vi "ZCP filiter.vi"(2 "Cutoff Frequency":i32=100, 3 "Sampling Frequency":i32=200000, 4 "Noise Band":dbl=-2.0, 5 "Data":dbl[](array[numeric])) -> (0 "Filiter Voltage":dbl[](array[numeric]), 1 "ZCP":i32[](array[numeric]))   [LabVIEW 2013]
uses:
  <vilib>/ptbypt/NI_PtbyPt.lvlib
panel:
  out "Waveform Graph":dbl[][](graph)
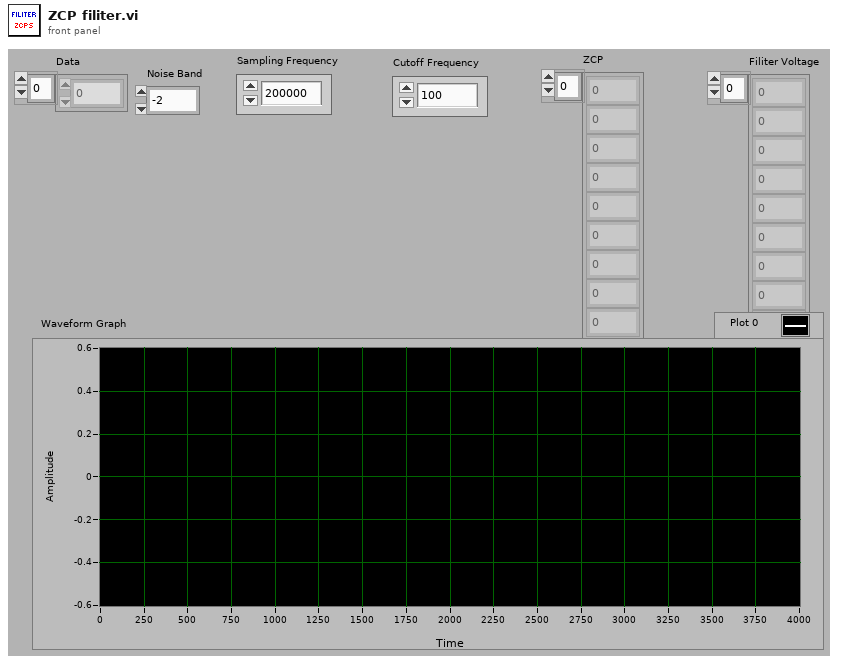
[diagram p1: front panel]
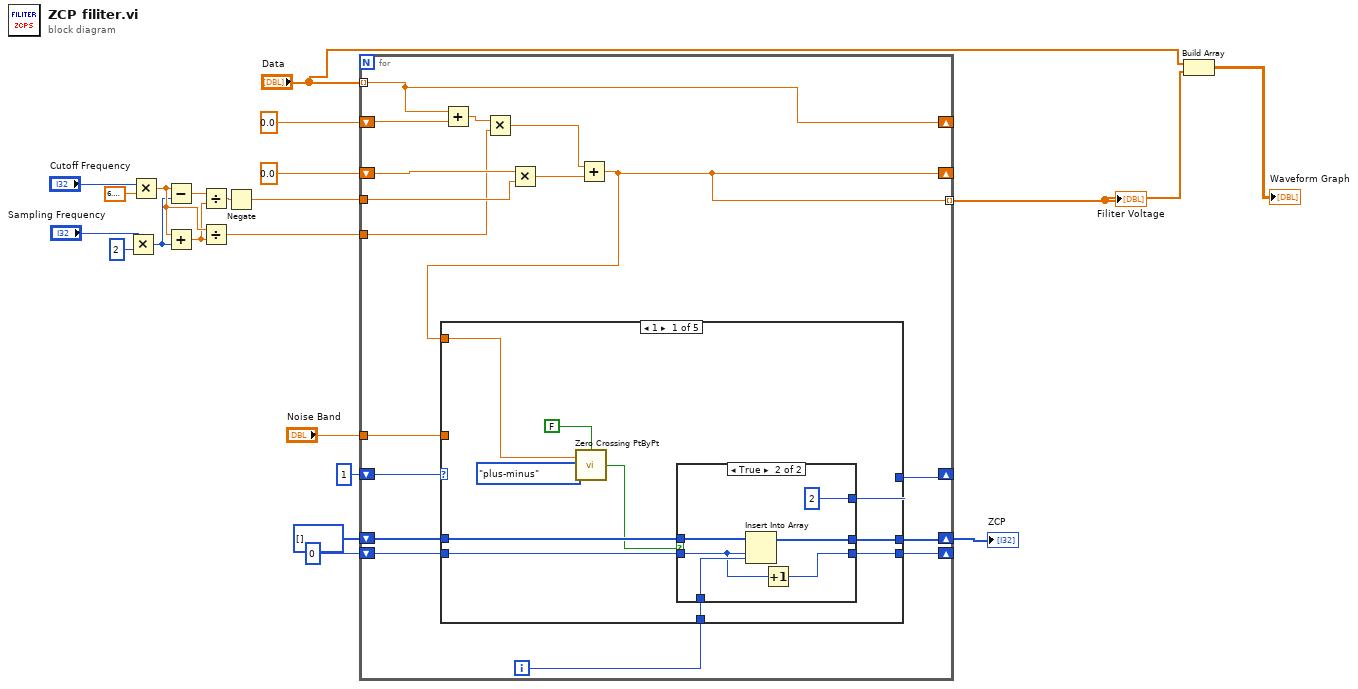
[diagram p0: block diagram]
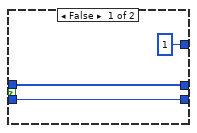
[diagram p2: hidden frame]
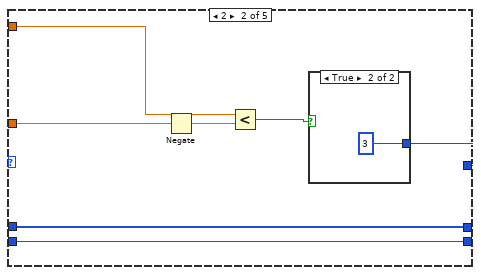
[diagram p3: hidden frame]
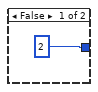
[diagram p4: hidden frame]
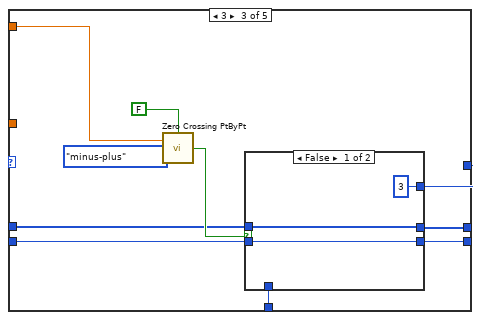
[diagram p5: hidden frame]
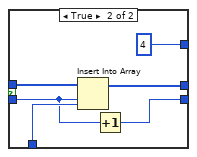
[diagram p6: hidden frame]
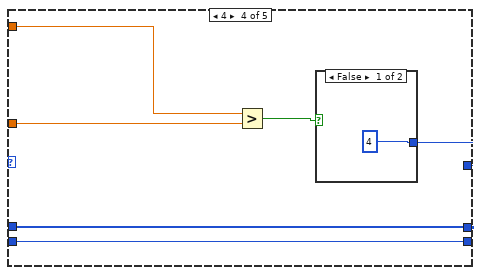
[diagram p7: hidden frame]
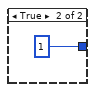
[diagram p8: hidden frame]
diagram:
  n1 = Multiply(x="Sampling Frequency", y=i16 2) -> (x*y=w13:i32)
  n2 = Multiply(x="Cutoff Frequency", y=6.283185307179586) -> (x*y=w14:dbl)
  n3 = Subtract(x=w14, y=w13) -> (x-y=w12:dbl)
  n4 = Add(x=w14, y=w13) -> (x+y=w11:dbl)
  n5 = Divide(x=w12, y=w11) -> (x/y=w8:dbl)
  n6 = Divide(x=w14, y=w11) -> (x/y=w6:dbl)
  n7 = Negate(x=w8) -> (-x=w7:dbl)
  n8 = for {
    shift-right: [w37] -> _
    shift-left: 1 -> [w38]
    tunnel: "Data" -> [w23] mode=indexing
    shift-right: [w34] -> w20
    shift-left: i32[] [] -> [w35]
    shift-right: [w32] -> _
    shift-left: 0 -> [w33]
    tunnel: "Noise Band" -> [w31]
    shift-right: [w23] -> _
    shift-left: 0.0 -> [w30]
    shift-right: [w22] -> _
    shift-left: 0.0 -> [w28]
    tunnel: w7 -> [w27]
    tunnel: w6 -> [w26]
    tunnel: [w22] -> w2 mode=indexing
    i -> [w36]
    n9 = Add(x=w23, y=w30) -> (x+y=w29:dbl)
    n10 = Multiply(x=w29, y=w26) -> (x*y=w25:dbl)
    n11 = Multiply(x=w28, y=w27) -> (x*y=w24:dbl)
    n12 = Add(x=w25, y=w24) -> (x+y=w22:dbl)
    n13 = case shown="1" w38 {
      tunnel: [w39 w60 w67 w87 _] -> w37
      tunnel: w22 -> [w47 w62 w74 w88 _]
      tunnel: w36 -> [w43 _ w68 _ _]
      tunnel: w35 -> [w45 w64 w72 w91 w95]
      tunnel: [w44 w64 w70 w91 w95] -> w34
      tunnel: w33 -> [w42 w63 w71 w90 w94]
      tunnel: [w40 w63 w69 w90 w94] -> w32
      tunnel: w31 -> [_ w59 _ w86 _]
      frame 1 {
        n14 = call <vilib>:"Zero Crossing PtByPt.vi"("initialize"=FALSE, "direction"=enum16{"either", "minus-plus", "plus-minus"}."plus-minus", "input data point"=w47) -> ("crossing"=w41:bool)
        n15 = case shown="True" w41 {
          tunnel: w45 -> [w51 w57]
          tunnel: [w51 w56] -> w44
          tunnel: w43 -> [_ w55]
          tunnel: w42 -> [w50 w54]
          tunnel: [w50 w53] -> w40
          tunnel: [1 2] -> w39
          frame False {
          }
          frame True {
            n16 = Insert Into Array(array=w57, index=w54, new element=w55) -> (w56:i32[])
            n17 = Increment(x=w54) -> (x+1=w53:i32)
          }
        }
      }
      frame 2 {
        n18 = Negate(x=w59) -> (-x=w58:dbl)
        n19 = Less?(x=w62, y=w58) -> (x < y?=w61:bool)
        n20 = case shown="True" w61 {
          tunnel: [2 3] -> w60
          frame False {
          }
          frame True {
          }
        }
      }
      frame 3 {
        n21 = call <vilib>:"Zero Crossing PtByPt.vi"("initialize"=FALSE, "direction"=enum16{"either", "minus-plus", "plus-minus"}."minus-plus", "input data point"=w74) -> ("crossing"=w73:bool)
        n22 = case shown="False" w73 {
          tunnel: w72 -> [w79 w85]
          tunnel: [w79 w84] -> w70
          tunnel: w68 -> [_ w83]
          tunnel: w71 -> [w78 w82]
          tunnel: [w78 w81] -> w69
          tunnel: [3 4] -> w67
          frame False {
          }
          frame True {
            n23 = Insert Into Array(array=w85, index=w82, new element=w83) -> (w84:i32[])
            n24 = Increment(x=w82) -> (x+1=w81:i32)
          }
        }
      }
      frame 4 {
        n25 = Greater?(x=w88, y=w86) -> (0:w89:bool)
        n26 = case shown="False" w89 {
          tunnel: [4 1] -> w87
          frame False {
          }
          frame True {
          }
        }
      }
      frame Default {
      }
    }
  }
  "ZCP" <- w20
  "Filiter Voltage" <- w2
  n27 = Build Array("Data", w2) -> (→"Waveform Graph":dbl[][])
